vi "IsString.vi"(4 "Value String in":string) -> (0 "IsString":bool, 2 "String Value":string)   [LabVIEW 2016]
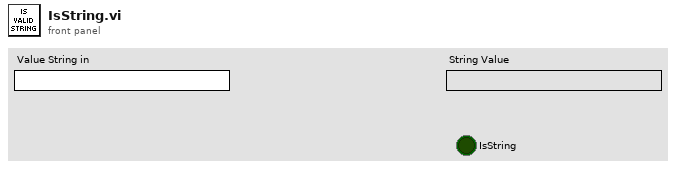
[diagram p1: front panel]
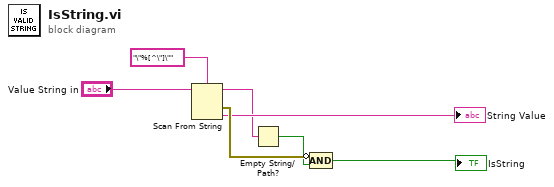
[diagram p0: block diagram]
diagram:
  n1 = Scan From String(format string="\"%[^\"]\"", input string="Value String in") -> (remaining string=w3:string, error out=w5:errorcluster, output 1=→"String Value":string)  [unwired: 3 in, 1 out]
  n2 = Empty String/Path?(string/path=w3) -> (empty?=w2:bool)
  n3 = Compound Arithmetic op=AND(invert w5, w2) -> (→"IsString":bool)
